vi "U8_3_byte_Array_to_graph.vi"(10 "Array In":u8[](array[numeric]), 11 "Nmbr_of_datasamples":dbl=128.0) -> (1 "mV":dbl, 2 "Waveform Graph":dbl[](graph), 3 "Loop count":dbl)   [LabVIEW 2012]
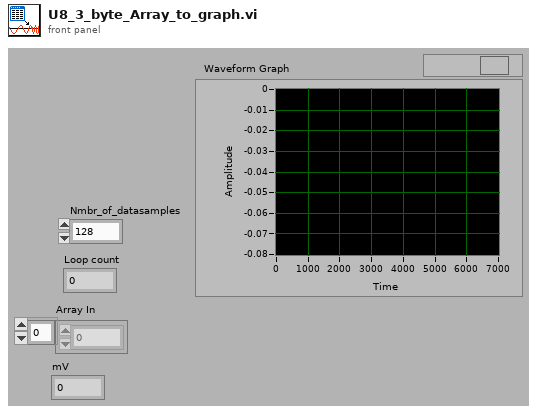
[diagram p1: front panel]
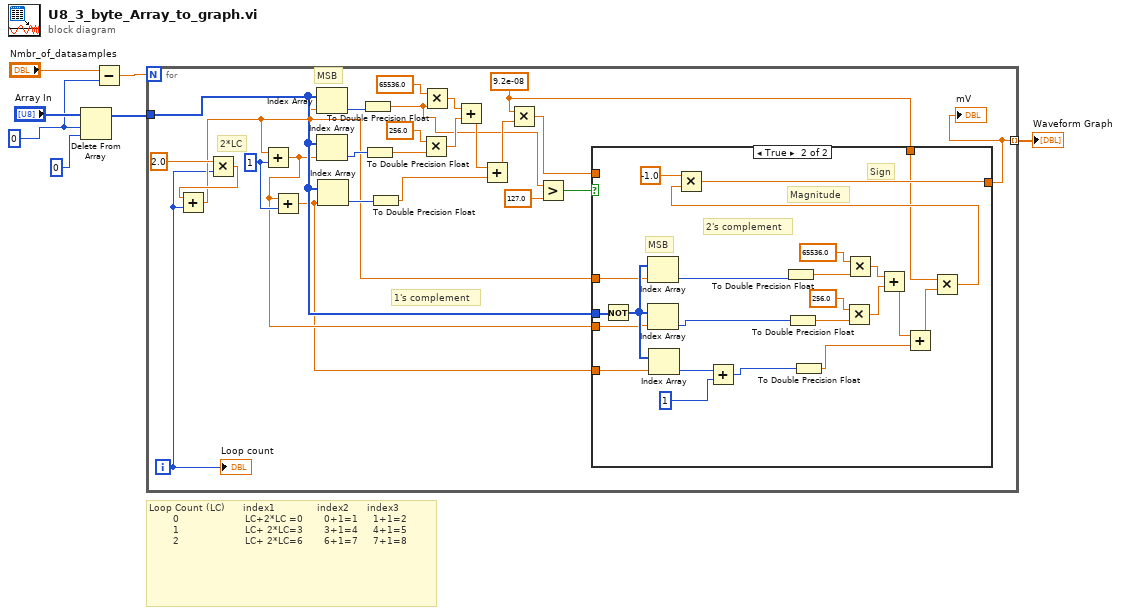
[diagram p0: block diagram]
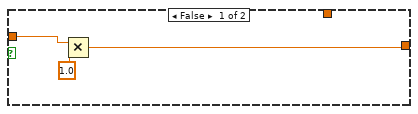
[diagram p2: hidden frame]
diagram:
  w2 = 0
  # "Loop Count (LC)      index1              index2      index3      \n        0                      LC+2*LC =0       0+1=1     1+1=2\n        1                      LC+ 2*LC=3       3+1=4     4+1=5\n        2                      LC+ 2*LC=6       6+1=7     7+1=8"
  n1 = Delete From Array(array="Array In", length=w2, index=0) -> (array with subset deleted=w1:u8[])  [unwired: 1 out]
  n2 = Subtract(x="Nmbr_of_datasamples", y=w2) -> (x-y=w4:dbl)
  n3 = for {
    N: w4 -> [_]
    tunnel: [w10] -> w7 mode=indexing
    tunnel: w1 -> [w14]
    i -> [w9]
    w8 = 9.2e-08
    w24 = 1
    # "1's complement"
    # "MSB"
    # "2*LC"
    n4 = Multiply(x=2.0, y=w9) -> (x*y=w22:dbl)
    n5 = Add(x=w22, y=w9) -> (x+y=w13:dbl)
    n6 = Add(x=w13, y=w24) -> (x+y=w12:dbl)
    n7 = Add(x=w12, y=w24) -> (x+y=w11:dbl)
    n8 = Index Array(array=w14, index=w13) -> (element=w17:u8)
    n9 = Index Array(array=w14, index=w12) -> (element=w16:u8)
    n10 = Index Array(array=w14, index=w11) -> (element=w15:u8)
    n11 = To Double Precision Float(number=w17) -> (double precision float=w18:dbl)
    n12 = To Double Precision Float(number=w16) -> (double precision float=w30:dbl)
    n13 = To Double Precision Float(number=w15) -> (double precision float=w26:dbl)
    n14 = Multiply(x=256.0, y=w30) -> (x*y=w28:dbl)
    n15 = Multiply(x=65536.0, y=w18) -> (x*y=w32:dbl)
    n16 = Add(x=w32, y=w28) -> (x+y=w27:dbl)
    n17 = Add(x=w27, y=w26) -> (x+y=w25:dbl)
    n18 = Multiply(x=w8, y=w25) -> (x*y=w21:dbl)
    n19 = Greater?(x=w18, y=127.0) -> (0:w20:bool)
    n20 = case shown="True" w20 {
      tunnel: [w35 w58] -> w10
      tunnel: w21 -> [w34 _]
      tunnel: w14 -> [_ w45]
      tunnel: w13 -> [_ w40]
      tunnel: w12 -> [_ w39]
      tunnel: w11 -> [_ w38]
      tunnel: w8 -> [_ w36]
      frame False {
        n21 = Multiply(x=w34, y=1.0) -> (x*y=w35:dbl)
      }
      frame True {
        # "Magnitude"
        # "Sign"
        # "2's complement"
        # "MSB"
        n22 = Not(x=w45) -> (.not. x?=w44:u8[])
        n23 = Index Array(array=w44, index=w40) -> (element=w47:u8)
        n24 = Index Array(array=w44, index=w39) -> (element=w46:u8)
        n25 = Index Array(array=w44, index=w38) -> (element=w43:u8)
        n26 = Add(x=w43, y=1) -> (x+y=w41:i32)
        n27 = To Double Precision Float(number=w47) -> (double precision float=w48:dbl)
        n28 = To Double Precision Float(number=w46) -> (double precision float=w54:dbl)
        n29 = To Double Precision Float(number=w41) -> (double precision float=w50:dbl)
        n30 = Multiply(x=256.0, y=w54) -> (x*y=w52:dbl)
        n31 = Multiply(x=65536.0, y=w48) -> (x*y=w56:dbl)
        n32 = Add(x=w56, y=w52) -> (x+y=w51:dbl)
        n33 = Add(x=w51, y=w50) -> (x+y=w49:dbl)
        n34 = Multiply(x=w36, y=w49) -> (x*y=w37:dbl)
        n35 = Multiply(x=-1.0, y=w37) -> (x*y=w58:dbl)
      }
    }
    "mV" <- w10
    "Loop count" <- w9
  }
  "Waveform Graph" <- w7
